vi "SimpleGetSpectrum.vi"(8 "Error In":errorcluster, 10 "Channel":u8=1 min=1 max=16 step=1, 11 "Address":string="10.0.0.55") -> (0 "Error Out":errorcluster, 1 "SN":u64, 2 "Time Stamp (ns)":u64, 3 "Spectrum Graph":cluster{dbl[], "Spectrum, db":dbl[]}[](graph))   [LabVIEW 2019]
doc: "This example VI demonstrates the use of the #GetSpectrum command to retrieve spectral data from Hyperion instruments.s"
uses:
  h.Library/COMM/CTL/h.COMM.Socket Type.ctl
  h.Library.lvlib
panel:
  # "Hyperion Simple #GetSpectrum Example"
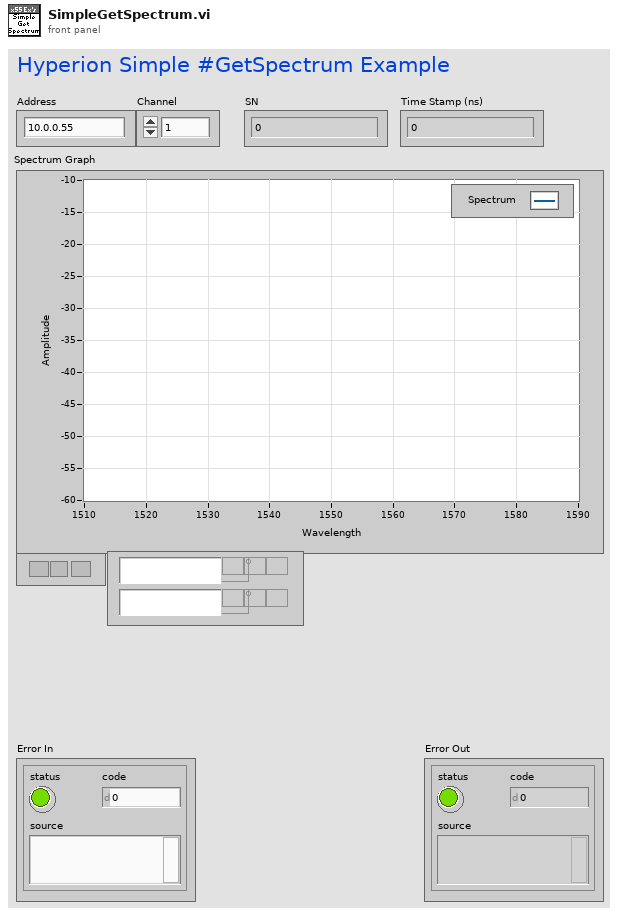
[diagram p1: front panel]
types:
  T1 = typedef "h.Library.lvlib/h.COMM.Socket Type.ctl" = u16
  T2 = typedef "h.Library.lvlib/h.ACQ.SpectralData.ctl" = cluster{"Spectrum":T3[], "Start Wvl":dbl, "Wvl Inc":dbl, "SN":u64, "Time Stamp (ns)":u64}
  T3 = typedef "h.Library.lvlib/h.ACQ.Spectrum.ctl" = cluster{"Spectrum, db":dbl[]}
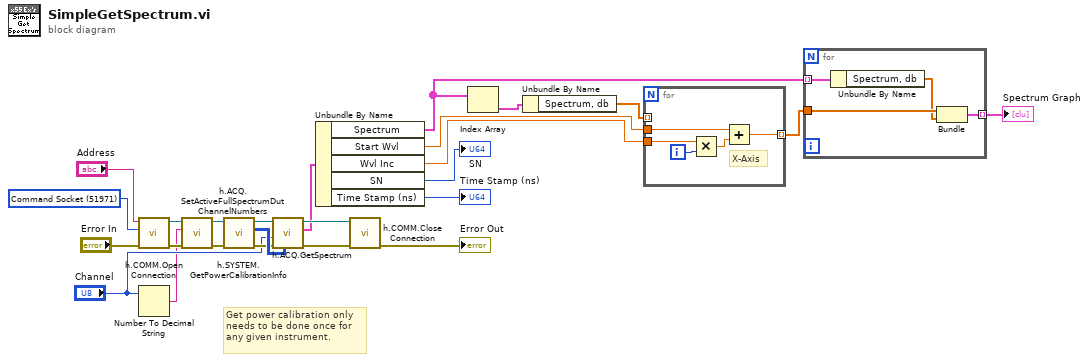
[diagram p0: block diagram]
diagram:
  w14 = T1 51971 items=["Command Socket"=51971, "Streaming Data Socket"=51972] ("Port")
  # "Get power calibration only\nneeds to be done once for\nany given instrument."
  n1 = call "h.COMM.Open Connection.vi"("error in"="Error In", "Port"=w14, "Address"="Address") -> ("error out"=w6:errorcluster, "Connection ID"=w5:refnum<k5>)  [unwired: 7 in]
  n2 = Number To Decimal String(number="Channel") -> (decimal integer string=w1:string)  [unwired: 1 in]
  n3 = call "h.ACQ.SetActiveFullSpectrumDutChannelNumbers.vi"("error in"=w6, "List of active channels (space delimited)"=w1, "Connection ID In"=w5) -> ("error out"=w3:errorcluster, "Connection ID Out"=w4:refnum<k5>)  [unwired: 7 in]
  n4 = call "h.SYSTEM.GetPowerCalibrationInfo.vi"("error in"=w3, "Connection ID"=w4) -> ("error out"=w11:errorcluster, "power scales and offsets"=w12:i32[][], "Connection ID out"=w13:refnum<k5>)  [unwired: 7 in]
  n5 = call "h.ACQ.GetSpectrum.vi"("power scales and offsets"=w12, "error in"=w11, "Single Channel"="Channel", "Connection ID In"=w13) -> ("error out"=w10:errorcluster, "Spectral Data"=w23:T2, "Connection ID Out"=w24:refnum<k5>)  [unwired: 5 in]
  n6 = Unbundle By Name(w23) -> ("Spectrum"=w18:T3[], "Start Wvl"=w22:dbl, "Wvl Inc"=w21:dbl, "SN"=→"SN":u64, "Time Stamp (ns)"=→"Time Stamp (ns)":u64)
  n7 = call "h.COMM.Close Connection.vi"("error in"=w10, "Connection ID"=w24) -> ("error out"=→"Error Out":errorcluster)  [unwired: 9 in]
  n8 = Index Array(array=w18) -> (element=w20:T3)  [unwired: 1 in]
  n9 = Unbundle By Name(w20) -> ("Spectrum, db"=w19:dbl[])
  n10 = for {
    tunnel: w22 -> [w28]
    tunnel: w21 -> [w30]
    tunnel: [w26] -> w17 mode=indexing
    tunnel: w19 -> [_] mode=indexing
    i -> [w29]
    # "X-Axis"
    n11 = Multiply(x=w30, y=w29) -> (x*y=w27:dbl)
    n12 = Add(x=w28, y=w27) -> (x+y=w26:dbl)
  }
  n13 = for {
    tunnel: w18 -> [w34] mode=indexing
    tunnel: w17 -> [w33]
    tunnel: [w31] -> w9 mode=indexing
    n14 = Unbundle By Name(w34) -> ("Spectrum, db"=w32:dbl[])
    n15 = Bundle(w33, "Spectrum, db"=w32) -> (w31:cluster{dbl[], "Spectrum, db":dbl[]})  [unwired: 1 in]
  }
  "Spectrum Graph" <- w9
